vi "Render.vi"(8 "error in (no error)":errorcluster, 10 "String in":string, 11 "Table in":refnum<class "Table.lvclass">) -> (0 "error out":errorcluster, 2 "String out":string, 3 "Table out":refnum<class "Table.lvclass">)   [LabVIEW 2021, in "LvMarkdown.lvlib" / "Table.lvclass"]
uses:
  Table.lvclass
  Table.lvclass/Table.ctl
  GetTableRow.vi
  GetHeader.vi
  Collection/GetElements.vi
  Collection/Collection.lvclass
  IRenderable/IRenderable.lvclass
  Alignment/Alignment.lvclass
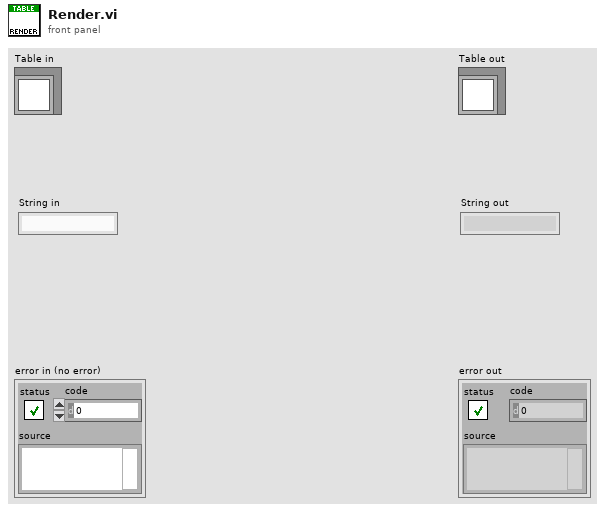
[diagram p1: front panel]
types:
  T1 = typedef "LvMarkdown.lvlib/Alignment.lvclass/AlignmentEnum.ctl" = enum16{"Left", "Center", "Right"}
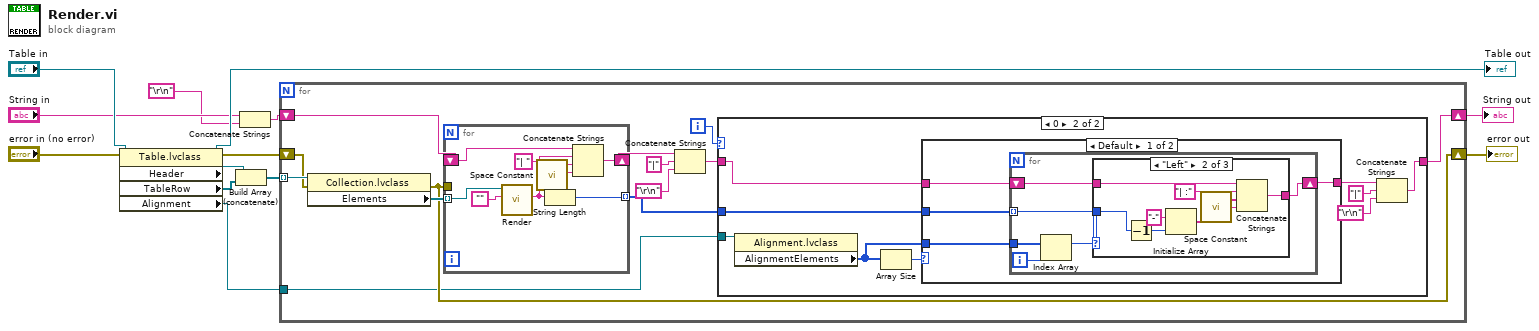
[diagram p0: block diagram]
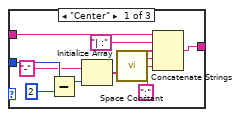
[diagram p3: hidden frame]
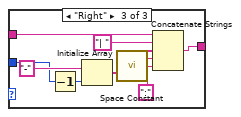
[diagram p4: hidden frame]
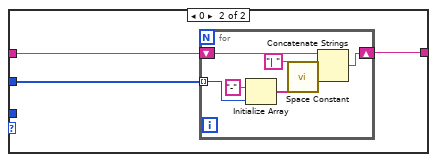
[diagram p5: hidden frame]
diagram:
  n1 = property class="Table.lvclass"(reference="Table in", error in="error in (no error)") -> (reference out=→"Table out":refnum<class "Table.lvclass">, error out=w5:errorcluster, "Header"=w8:refnum<class "Collection.lvclass">, "TableRow"=w7:refnum<class "Collection.lvclass">[], "Alignment"=w1:refnum<class "Alignment.lvclass">)
  n2 = Build Array (concatenate)(w8, w7) -> (w6:refnum<class "Collection.lvclass">[])
  n3 = Concatenate Strings("String in", "\r\n") -> (w3:string)
  n4 = for {
    shift-right: [w20] -> w9
    shift-left: w3 -> [w26]
    tunnel: w6 -> [w18] mode=indexing
    shift-right: [w15] -> w4
    shift-left: w5 -> [w16]
    tunnel: w1 -> [w14]
    i -> [w19]
    n5 = property class="Collection.lvclass"(reference=w18, error in=w16) -> (error out=w15:errorcluster, "Elements"=w17:refnum<class "IRenderable.lvclass">[])  [unwired: 1 out]
    n6 = for {
      shift-right: [w86] -> w25
      shift-left: w26 -> [w91]
      tunnel: w17 -> [w89] mode=indexing
      tunnel: [w84] -> w22 mode=indexing
      tunnel: w15 -> [_]
      n7 = call-dynamic "Render.vi"("String in"="", "IRenderable in"=w89) -> ("String out"=w85:string)  [unwired: 7 in, 2 out]
      n8 = call <vilib>:"Space Constant.vi"() -> ("String"=w87:string)
      n9 = String Length(string=w85) -> (length=w84:i32)
      n10 = Concatenate Strings(w91, "| " ("string"), w85, w87) -> (w86:string)
    }
    n11 = Concatenate Strings(w25, "|" ("string"), "\r\n") -> (w21:string)
    n12 = case shown="0" w19 {
      tunnel: w22 -> [_ w36]
      tunnel: w21 -> [w27 w35]
      tunnel: [w27 w31] -> w20
      tunnel: w14 -> [_ w30]
      frame Default {
      }
      frame 0 {
        n13 = property class="Alignment.lvclass"(reference=w30) -> ("AlignmentElements"=w29:T1[])  [unwired: 1 in, 2 out]
        n14 = Array Size(array=w29) -> (size(s)=w28:i32)
        n15 = case shown="Default" w28 {
          tunnel: w36 -> [w40 w76]
          tunnel: w35 -> [w39 w75]
          tunnel: [w38 w74] -> w32
          tunnel: w29 -> [w37 _]
          frame Default {
            n16 = for {
              tunnel: w40 -> [w45] mode=indexing
              shift-right: [w44] -> w38
              shift-left: w39 -> [w46]
              tunnel: w37 -> [w43]
              i -> [w41]
              n17 = Index Array(array=w43, index=w41) -> (element=w42:T1)
              n18 = case shown="\"Left\"" w42 {
                tunnel: w46 -> [w56 w64 w73]
                tunnel: w45 -> [w54 w62 w66]
                tunnel: [w50 w58 w68] -> w44
                frame "Center" {
                  n19 = Subtract(x=w54, y=2) -> (x-y=w49:i32)
                  n20 = Initialize Array("-", w49) -> (w52:string[])
                  n21 = call <vilib>:"Space Constant.vi"() -> ("String"=w51:string)
                  n22 = Concatenate Strings(w56, "| :" ("string"), w52, ":", w51) -> (w50:string)
                }
                frame "Left" {
                  n23 = Decrement(x=w62) -> (x-1=w57:i32)
                  n24 = Initialize Array("-", w57) -> (w60:string[])
                  n25 = call <vilib>:"Space Constant.vi"() -> ("String"=w59:string)
                  n26 = Concatenate Strings(w64, "| :" ("string"), w60, w59) -> (w58:string)
                }
                frame "Right" {
                  n27 = Decrement(x=w66) -> (x-1=w65:i32)
                  n28 = Initialize Array("-", w65) -> (w70:string[])
                  n29 = call <vilib>:"Space Constant.vi"() -> ("String"=w69:string)
                  n30 = Concatenate Strings(w73, "| " ("string"), w70, ":", w69) -> (w68:string)
                }
              }
            }
          }
          frame 0 {
            n31 = for {
              tunnel: w76 -> [w82] mode=indexing
              shift-right: [w81] -> w74
              shift-left: w75 -> [w83]
              n32 = Initialize Array("-", w82) -> (w78:string[])
              n33 = call <vilib>:"Space Constant.vi"() -> ("String"=w77:string)
              n34 = Concatenate Strings(w83, "| " ("string"), w78, w77) -> (w81:string)
            }
          }
        }
        n35 = Concatenate Strings(w32, "|" ("string"), "\r\n") -> (w31:string)
      }
    }
  }
  "error out" <- w4
  "String out" <- w9
